vi "TEST_L0_SUM_(1ST)_NEW.vi"(7 "Serial Number":string="SN_00187", 8 "error in (no error)":errorcluster, 11 "Instrument VISA in":T1={"AWG VISA"="AgilentGen1", "Oscilloscope  VISA "="AgilentOsc", "Integration Board IP"="172.16.17.47", "connection ID"=refnum, "report out"=refnum, "report file path"=path "C:/Users/omartinez/Desktop/L0nL1_Results"}) -> (0 "error out":errorcluster, 3 "Instrument VISA out":T1={"AWG VISA"="AgilentGen1", "Oscilloscope  VISA "="AgilentOsc", "Integration Board IP"="172.16.17.47", "connection ID"=refnum, "report out"=refnum, "report file path"=path "C:/Users/omartinez/Desktop/L0nL1_Results"})   [LabVIEW 2012]
uses:
  <vilib>/Utility/NIReport.llb/NI_report.lvclass
  <vilib>/Utility/NIReport.llb/HTML/NI_HTML.lvclass
  <instrlib>/Agilent 8000 Series/Public/Configure/Configure Math (Binary Operation).vi
  Sum_Abrilader/L0_Sum_Adder Folder/C/Program Files/National Instruments/LabVIEW 2012/instr.lib/Agilent 8000 Series/Public/Data/Low Level/Fetch Measurement (More).vi
  <instrlib>/Agilent 8000 Series/Agilent 8000 Series.lvlib
panel:
  in  "Amp Scaler":dbl=1.0
  in  "Clip Select":i32[](array[numeric])=[1, 2, 3]
  in  "Atenuation":i32[](array[numeric])=[0, 15]
  in  "IB_Clip":i32[](array[numeric])=[7, 23, 31, 63]
  in  "Voltages":dbl[](array[numeric])=[0.05, 0.1, 0.2, 0.5, 0.8]
  in  "Channels":i32[](array[numeric])=[0, 1, 2, 3, 4, 5, 6]
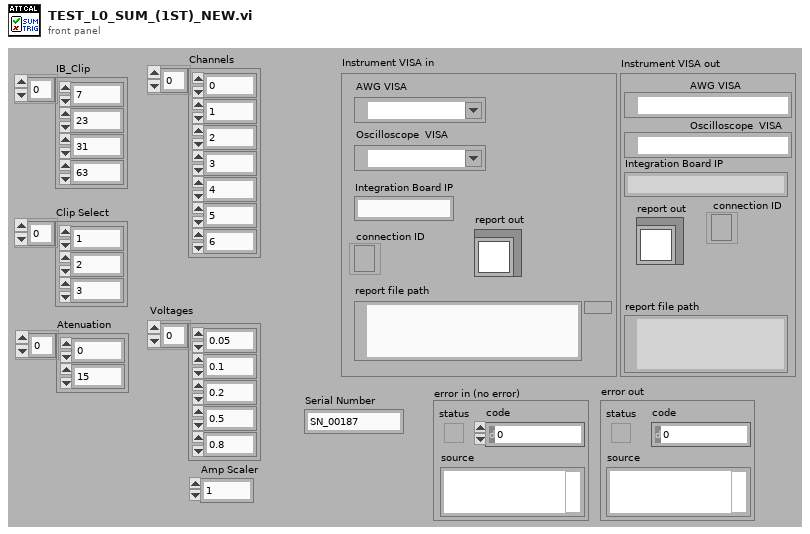
[diagram p1: front panel]
types:
  T1 = cluster{"AWG VISA":refnum<visa-resource-name>, "Oscilloscope  VISA ":refnum<visa-resource-name>, "Integration Board IP":string, "connection ID":refnum<k5>, "report out":refnum<class "NI_report.lvclass">, "report file path":path}
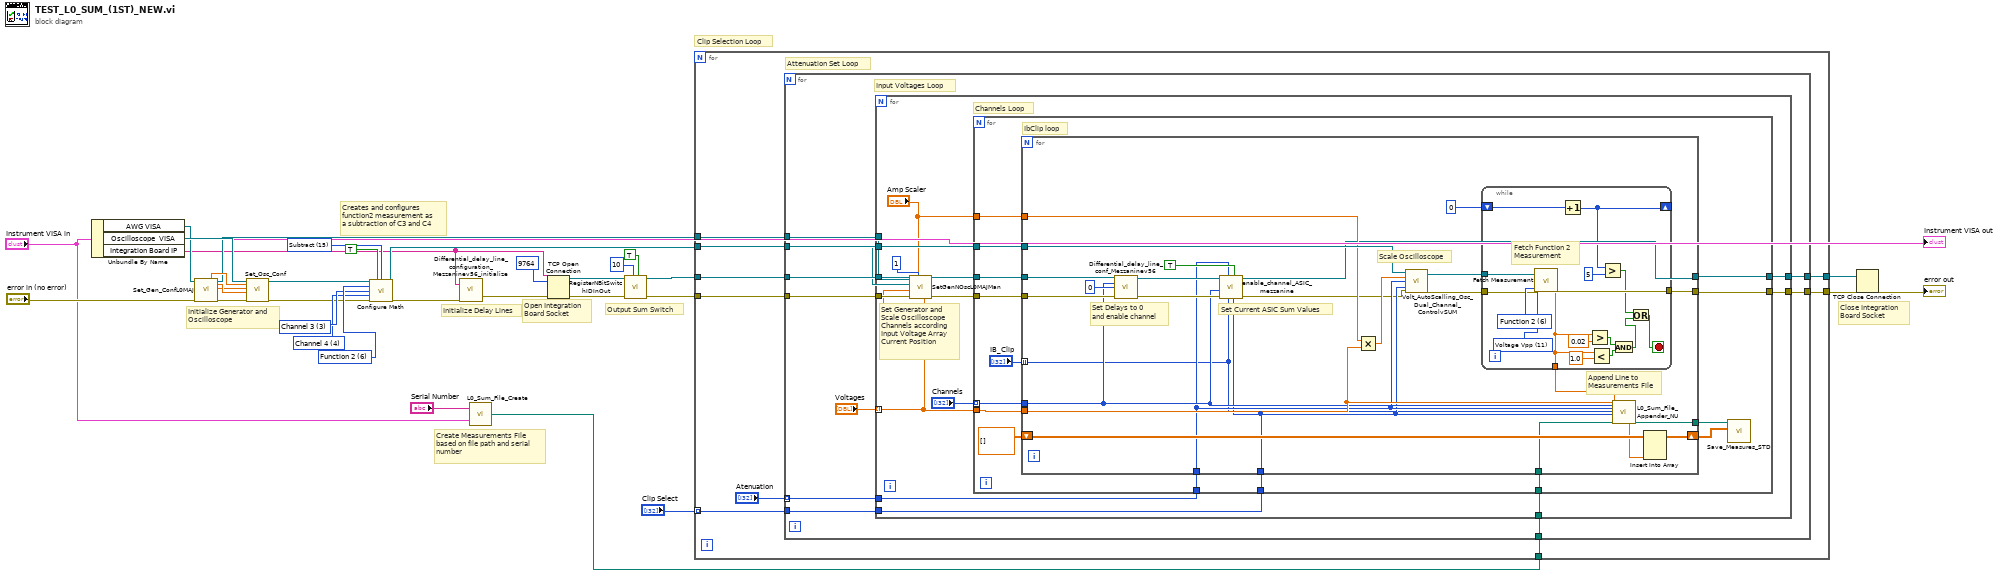
[diagram p0: block diagram]
diagram:
  w11 = u16 6 items=["Function 1"=5, "Function 2"=6, "Function 3"=7, "Function 4"=8] ("Math Channel (5: Function 1)")
  w12 = u16 15 items=["Add"=12, "Divide"=13, "Multiply"=14, "Subtract"=15, "Common Mode"=16, "Versus"=17] ("Math Operation (12: Add)")
  w10 = 3 items=["Channel 1"=1, "Channel 2"=2, "Channel 3"=3, "Channel 4"=4] ("Channel (1: Channel 1)")
  w9 = 4 items=["Channel 1"=1, "Channel 2"=2, "Channel 3"=3, "Channel 4"=4] ("Channel (1: Channel 1)")
  # "Clip Selection Loop"
  # "Create Measurements File\nbased on file path and serial\nnumber"
  # "Close Integration \nBoard Socket"
  # "Output Sum Switch"
  # "Open Integration\nBoard Socket"
  # "Initialize Delay Lines"
  # "Initialize Generator and \nOscilloscope"
  # "Creates and configures\nfunction2 measurement as\na subtraction of C3 and C4"
  n1 = Unbundle By Name("Instrument VISA in") -> ("AWG VISA"=w29:refnum<visa-resource-name>, "Oscilloscope  VISA"=w30:refnum<visa-resource-name>, "Integration Board IP"=w1:string)
  n2 = call "Set_Gen_ConfL0MAJ.vi"("AWG VISA"=w29, "error in (no error)"="error in (no error)") -> ("Amplitude 1 OUT"=w27:dbl, "VISA resource name out"=w21:refnum<visa-resource-name>, "Pulse Width in seconds 1 OUT"=w26:dbl, "Trigger Level 1"=w25:dbl, "error out"=w31:errorcluster)  [unwired: 10 in, 3 out]
  n3 = call "Set_Osc_Conf.vi"("VISA resource name"=w30, "Amplitude IN"=w27, "Trigger Level IN"=w25, "Pulse Width in seconds IN"=w26, "error in (no error)"=w31) -> ("VISA resource name out"=w8:refnum<visa-resource-name>, "error out"=w7:errorcluster)  [unwired: 13 in]
  n4 = call-poly <instrlib>:"Configure Math.vi"("VISA resource name"=w8, "Enable Math Channel (T:Enable)"=TRUE, "Math Operation (12: Add)"=w12, "Math Channel (5: Function 1)"=w11, "Math Operand (1: Channel 1)"=w10, "Math Operand (2: Channel 2)"=w9, "error in (no error)"=w7) -> ("VISA resource name out"=w5:refnum<visa-resource-name>, "error out"=w6:errorcluster)  [unwired: 7 in]
  n5 = call "Differential_delay_line_configuration_Mezzaninev56_initialize.vi"("error in (no error)"=w6, "address"=w1) -> ("error out 2"=w24:errorcluster)
  n6 = call "L0_Sum_File_Create.vi"("input cluster"="Instrument VISA in", "Serial Number"="Serial Number") -> ("appended path"=w2:path)
  n7 = TCP Open Connection(address=w1, remote port or service name=9764, error in (no error)=w24) -> (connection ID=w19:refnum<k5>, error out=w23:errorcluster)  [unwired: 2 in]
  n8 = call "RegisterNBitSwitchIDInOut.vi"("Switch Bit"=TRUE, "N Bit"=10, "error in (no error)"=w23, "connection ID"=w19) -> ("error out"=w20:errorcluster, "connection ID out"=w18:refnum<k5>)  [unwired: 5 in]
  n9 = for {
    tunnel: w20 -> [w39]
    tunnel: [w40] -> w22
    tunnel: w18 -> [w42]
    tunnel: [w41] -> w14
    tunnel: w5 -> [w38]
    tunnel: w21 -> [w37]
    tunnel: "Clip Select" -> [w34] mode=indexing
    tunnel: w2 -> [w35]
    # "Attenuation Set Loop"
    n10 = for {
      tunnel: w42 -> [w52]
      tunnel: [w51] -> w41
      tunnel: [w50] -> w40
      tunnel: w39 -> [w49]
      tunnel: w38 -> [w48]
      tunnel: w37 -> [w47]
      tunnel: w34 -> [w46]
      tunnel: "Atenuation" -> [w43] mode=indexing
      tunnel: w35 -> [w44]
      # "Input Voltages Loop"
      n11 = for {
        tunnel: w52 -> [w66]
        tunnel: [w65] -> w51
        tunnel: [w64] -> w50
        tunnel: w49 -> [w63]
        tunnel: w48 -> [w56]
        tunnel: w47 -> [w60]
        tunnel: w46 -> [w59]
        tunnel: w43 -> [w58]
        tunnel: "Voltages" -> [w53] mode=indexing
        tunnel: w44 -> [w55]
        # "Channels Loop"
        # "Set Generator and\nScale Oscilloscope\nChannels according\nInput Voltage Array\nCurrent Position"
        n12 = call "SetGenNOscL0MAJMan.vi"("Input Voltage"=w53, "Amp Scaler"="Amp Scaler", "NChannels"=1, "error in (no error)"=w63, "Output Voltage"=w53, "VISA resource name"=w56, "AWG VISA"=w60) -> ("error out 2"=w62:errorcluster)  [unwired: 4 in]
        n13 = for {
          tunnel: w66 -> [w81]
          tunnel: [w80] -> w65
          tunnel: [w79] -> w64
          tunnel: w62 -> [w78]
          tunnel: w59 -> [w77]
          tunnel: w58 -> [w76]
          tunnel: "Channels" -> [w67] mode=indexing
          tunnel: w56 -> [w74]
          tunnel: w53 -> [w73]
          tunnel: w55 -> [w72]
          tunnel: "Amp Scaler" -> [w68]
          # "IbClip loop"
          n14 = for {
            tunnel: w81 -> [w106]
            tunnel: [w84] -> w80
            tunnel: [w101] -> w79
            tunnel: w78 -> [w104]
            tunnel: w77 -> [w87]
            tunnel: w76 -> [w88]
            tunnel: w67 -> [w90]
            tunnel: "IB_Clip" -> [w82] mode=indexing
            tunnel: w74 -> [w99]
            tunnel: w73 -> [w92]
            tunnel: w72 -> [w91]
            shift-right: [w96] -> w69
            shift-left: dbl[][] [] ("Y") -> [w97]
            tunnel: [w94] -> w70
            tunnel: w68 -> [w93]
            # "Scale Oscilloscope"
            # "Set Current ASIC Sum Values"
            # "Append Line to \nMeasurements File"
            # "Set Delays to 0 \nand enable channel"
            n15 = call "Differential_delay_line_conf_Mezzaninev56.vi"("connection ID"=w106, "channel"=w90, "Delay value"=u16 0, "error in (no error)"=w104) -> ("connection ID out"=w105:refnum<k5>, "error out 2"=w107:errorcluster)  [unwired: 4 in, 6 out]
            n16 = call "enable_channel_ASIC_mezzanine.vi"("Clip_sel_b"=w87, "maj/sum"=TRUE, "Ib_clipVb"=w82, "Att gain"=w88, "error in"=w107, "Channel"=w90, "connection ID"=w105) -> ("error out"=w85:errorcluster, "connection ID out"=w84:refnum<k5>)  [unwired: 2 in, 1 out]
            n17 = Multiply(x=w93, y=w92) -> (x*y=w95:dbl)
            n18 = call "Volt_AutoScalling_Osc_Dual_Channel_ControlvSUM.vi"("VISA Oscilloscope"=w99, "Voltage In"=w95, "Att"=w88, "Clip"=w87, "error in"=w85) -> ("VISA resource name out"=w98:refnum<visa-resource-name>, "error out"=w100:errorcluster)  [unwired: 9 in]
            n19 = while {
              tunnel: [w121] -> w101
              tunnel: w100 -> [w120]
              tunnel: w98 -> [w119]
              tunnel: [w116] -> w86
              shift-right: [w112] -> _
              shift-left: u16 0 ("Delay value") -> [w113]
              stop <- w109 stop-if-true
              w123 = 11 items=["Rise Time", "Fall Time", "Frequency", "Period", "Voltage RMS(AC)", "Voltage RMS(DC)", "Voltage RMS (AC,cycle)", "Voltage RMS (DC,cycle)", "Voltage Max", "Voltage Min", "Voltage Middle", "Voltage Vpp", "Voltage High", "Voltage Low", "Voltage Average", "Voltage Average (cycle)", "Width Negative", "Width Positive", "Duty Cycle Positive", "Amplitude", "Overshoot", "Preshoot", "Voltage Base", "Voltage Upper", "Time Max", "Time Min", "Color Grade Crossing", "Color Grade Eye Width", "Color Grade Eye Height", "Color Grade Eye Q-Factory", "Color Grade Eye Duty Cycle Distortion(Percent)", "Color Grade Eye Duty Cycle Distortion(Time)", "Color Grade Eye Jitter(PP)", "Color Grade Eye Width(RMS)", "Cycle-cycle Duty Jitter(Rising)", "Cycle-cycle Duty Jitter(Falling)", "Cycle-cycle Jitter(Rising)", "Cycle-cycle Jitter(Falling)", "Cycle-cycle - Width", "Cycle-cycle + Width", "Date Rate", "Unit Interval", "FFT Delta Frequency", "FFT Delta Magnitude", "FFT Frequency", "FFT Magnitude", "Slew Rate", "Area (Entire Display)", "Area(Single Cycle)", "Duty Cycle (Rising)", "Duty Cycle (Falling)"] ("Measurement Function (0: Rise Time)")
              w122 = 6 items=["Channel 1"=1, "Channel 2"=2, "Channel 3"=3, "Channel 4"=4, "Function 1"=5, "Function 2"=6, "Function 3"=7, "Function 4"=8, "Memory 1"=9, "Memory 2"=10, "Memory 3"=11, "Memory 4"=12] ("Channel (1: Channel 1)")
              # "Fetch Function 2\nMeasurement"
              n20 = call-poly "Fetch Measurement.vi"("VISA resource name"=w119, "Channel (1: Channel 1)"=w122, "Measurement Function (0: Rise Time)"=w123, "error in (no error)"=w120) -> ("Measurement"=w116:dbl, "error out"=w121:errorcluster)  [unwired: 9 in, 1 out]
              n21 = Increment(x=w113) -> (x+1=w112:u16)
              n22 = Greater?(x=w116, y=0.02) -> (0:w118:bool)
              n23 = Less?(x=w116, y=1.0) -> (x < y?=w114:bool)
              n24 = Greater?(x=w112, y=u16 5) -> (0:w108:bool)
              n25 = And(x=w118, y=w114) -> (x .and. y?=w110:bool)
              n26 = Or(x=w108, y=w110) -> (x .or. y?=w109:bool)
            }
            n27 = call "L0_Sum_File_Appender_NU.vi"("Vin"=w92, "CH"=w90, "Att"=w88, "IbClip"=w82, "Clip"=w87, "Vmeas"=w86, "file path"=w91) -> ("appended array"=w89:dbl[], "file path 2"=w94:path)  [unwired: 19 in]
            n28 = Insert Into Array(array=w97, new element=w89) -> (w96:dbl[][])  [unwired: 2 in]
          }
          n29 = call "Save_Measures_STD.vi"("Data in"=w69, "file path (dialog if empty)"=w70) -> ()  [unwired: 10 in]
        }
      }
    }
  }
  n30 = TCP Close Connection(connection ID=w14, error in (no error)=w22) -> (error out=→"error out":errorcluster)  [unwired: 1 in, 1 out]
  "Instrument VISA out" <- "Instrument VISA in"
